vi "Cobra.vi"() -> ()   [LabVIEW 2020]
uses:
  <vilib>/High Genius/HG_WSI_Tookit/Dependencies/Library/IIC/IIC.lvclass
  C:/Program Files (x86)/National Instruments/LabVIEW 2020/vi.lib/High Genius/HG_WSI_Tookit/Dependencies/Library/HG_LIB/HG_LIB.lvclass
  <vilib>/Platform/TimedLoop/XDataNode/timing_clust.ctl
  <vilib>/Platform/TimedLoop/XDataNode/nitl_modes.ctl
  <vilib>/Platform/TimedLoop/XDataNode/wakeup.ctl
  <vilib>/platform/TimedLoop/XDataNode/XDataNode.xnode
  <vilib>/High Genius/HG_WSI_Tookit/Dependencies/Library/HG_LIB/HG_LIB.lvclass
  <vilib>/Platform/TimedLoop/XDataNode/XDNodeRunTimeDep.lvlib
panel:
  out "QTI":dbl[](array[numeric])
  in  "stop":bool
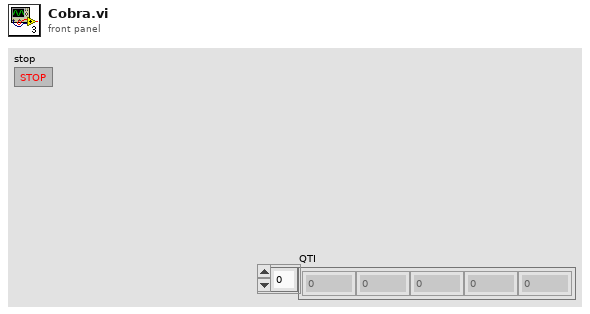
[diagram p1: front panel]
types:
  T1 = enum16{"DI", "DO", "AI", "Pulse", "PWM", "ISQ", "ENC", "CAN", "IIC", "IMU"}
  T2 = typedef "XDNodeRunTimeDep.lvlib/timing_clust.ctl" = cluster{"Expected End [f-1]":u64, "Actual End [f-1]":u64, "Finished Late? [f-1]":bool, "Expected End [i-1]":u64, "Actual End [i-1]":u64, "Finished Late? [i-1]":bool, "Expected Start [i]":u64, "Actual Start [i]":u64, "Expected Start [f]":u64, "Actual Start [f]":u64, "Source Name":string, "Structure Name":string, "Period":i64, "Deadline":i64, "Offset":i64, "Start":i64, "Priority":i32, "Timeout":i32, "Mode":T3, "Wakeup Reason":T4, "Error":errorcluster, "Source Type":string, "Secondary Source Type":string, "Global End Time":u64, "Global Start Time":u64, "Frame Duration":u64, "Iteration Duration":u64, "Assigned CPU":i32, "I/O Scan Engine Mode":u32}
  T3 = typedef "XDNodeRunTimeDep.lvlib/nitl_modes.ctl" = enum32{"No Change", "Process missed periods, maintain original phase", "Discard missed periods, maintain original phase", "Process missed periods, ignore original phase", "Discard missed periods, ignore original phase"}
  T4 = typedef "XDNodeRunTimeDep.lvlib/wakeup.ctl" = enum32{"Normal", "Aborted", "Asynchronous wakeup", "Timing source error", "Timed loop error", "Timeout"}
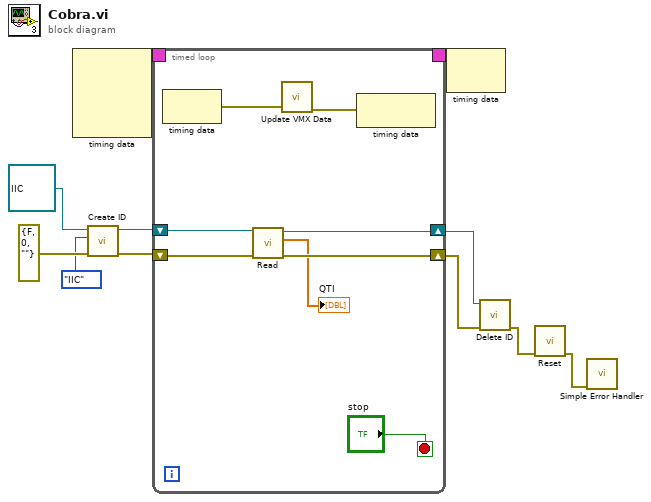
[diagram p0: block diagram]
diagram:
  n1 = node-c288() -> (w11:T2)  [unwired: 4 in]
  n2 = call <vilib>:"Create ID.vi"("error in (no error)"=errorcluster {"status"=FALSE, "code"=0, "source"=""}, "Function"=T1."IIC", "HG_LIB in"=refnum<class "IIC.lvclass"> refnum ("VMX Library.lvlib:IIC.lvclass")) -> ("error out"=w4:errorcluster, "HG_LIB out"=w5:refnum<class "IIC.lvclass">)  [unwired: 7 in]
  n3 = timed-loop {
    timing: w11 -> [_]
    timing-out: [_] -> w10
    shift-right: [w13] -> w2
    shift-left: w5 -> [w16]
    shift-right: [w14] -> w3
    shift-left: w4 -> [w15]
    stop <- "stop" stop-if-true
    n4 = node-c288() -> (w18:errorcluster)  [unwired: 1 in]
    n5 = call <vilib>:"Read.vi"("error in (no error)"=w15, "IIC in"=w16) -> ("error out"=w14:errorcluster, "QTI"=→"QTI":dbl[], "IIC out"=w13:refnum<class "IIC.lvclass">)  [unwired: 7 in]
    n6 = call <vilib>:"Update VMX Data.vi"("error in (no error)"=w18) -> ("error out"=w17:errorcluster)  [unwired: 10 in]
    n7 = node-c288(w17) -> ()  [unwired: 1 out]
  }
  n8 = node-c288(w10) -> ()  [unwired: 1 out]
  n9 = call <vilib>:"Delete ID.vi"("error in (no error)"=w3, "HG_LIB in"=w2) -> ("error out"=w9:errorcluster)  [unwired: 8 in, 1 out]
  n10 = call <vilib>:"Reset.vi"("error in (no error)"=w9) -> ("error out"=w8:errorcluster)  [unwired: 10 in]
  n11 = call <vilib>:"Simple Error Handler.vi"("error in (no error)"=w8) -> ()  [unwired: 4 in, 5 out]
